vi "DeCoF tuplerealbool query.vi"(4 "error in":errorcluster, 5 "use gsv":bool, 6 "param-name":string, 7 "Conncection ID in":T1) -> (0 "error out":errorcluster, 1 "boolean value":bool, 2 "real value":dbl, 3 "Conncection ID out":T1)   [LabVIEW 2013]
uses:
  subVIs/DeCoF connection.ctl
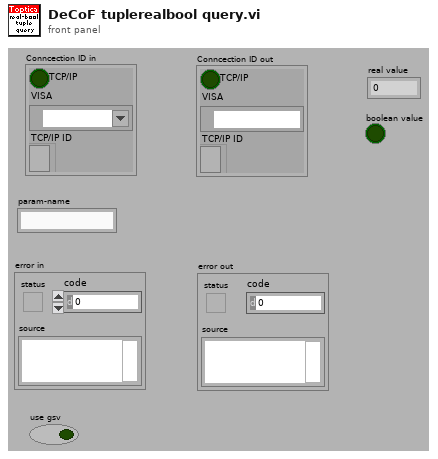
[diagram p1: front panel]
types:
  T1 = typedef "DeCoF connection.ctl" = cluster{"TCP/IP":bool, "VISA":refnum<visa-resource-name>, "TCP/IP ID":refnum<k5>}
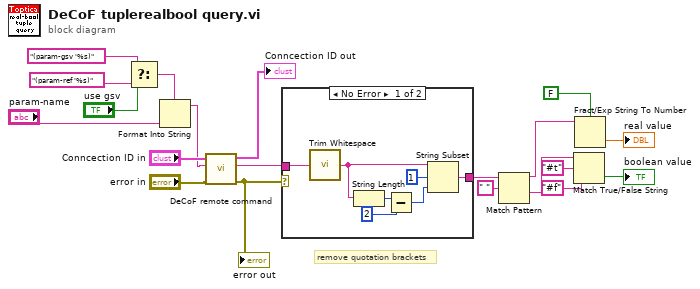
[diagram p0: block diagram]
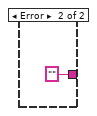
[diagram p2: hidden frame]
diagram:
  # "remove quotation brackets"
  n1 = Select(t="(param-gsv '%s)" ("format string"), s="use gsv", f="(param-ref '%s)" ("format string")) -> (s? t:f=w15:string)
  n2 = Format Into String(format string=w15, "param-name") -> (resulting string=w12:string)  [unwired: 2 in, 1 out]
  n3 = call "DeCoF remote command.vi"("error in (no error)"="error in", "command"=w12, "Conncection ID in"="Conncection ID in") -> ("error out"=w10:errorcluster, "answer string"=w11:string, "Conncection ID out"=→"Conncection ID out":T1)  [unwired: 2 in, 2 out]
  "error out" <- w10
  n4 = case shown="No Error" w10 {
    tunnel: w11 -> [w23 _]
    tunnel: [w21 "" ("trimmed string")] -> w5
    frame No Error {
      n5 = call <vilib>:"Trim Whitespace.vi"("string"=w23) -> ("trimmed string"=w26:string)  [unwired: 1 in]
      n6 = String Length(string=w26) -> (length=w24:i32)
      n7 = Subtract(x=w24, y=2) -> (x-y=w22:i32)
      n8 = String Subset(string=w26, offset (0)=1, length (rest)=w22) -> (substring=w21:string)
    }
    frame Error {
      (unwired) 0.0
      (unwired) FALSE ("selection")
    }
  }
  n9 = Match Pattern(string=w5, regular expression=" ") -> (before substring=w3:string, after substring=w7:string)  [unwired: 1 in, 2 out]
  n10 = Match True/False String(2:"#f" ("false string"), 3:"#t" ("true string"), 4:w7) -> (0:→"boolean value":bool)  [unwired: 1 out]
  n11 = Fract/Exp String To Number(use system decimal point (T)=FALSE, string=w3) -> (number=→"real value":dbl)  [unwired: 2 in, 1 out]
